vi "Clean Up Actor.vi"(8 "error in (no error)":errorcluster, 11 "Car Position Simulator in":refnum<class "Car Position Simulator.lvclass">) -> (0 "error out":errorcluster, 3 "Car Position Simulator out":refnum<class "Car Position Simulator.lvclass">)   [LabVIEW 2016, in "CLD Exam - Car Wash.lvlib" / "Car Position Simulator.lvclass"]
doc: "--\nCopyright © 2017 Composed SystemsI All rights reserved.\n\nAuthor: Jon McBee <jon.mcbee@composed.io>\n\nThis library is provided \"AS IS\" ,WITHOUT WARRANTIES OR\nCONDITIONS OF ANY KIND, either express or implied.\n\nComposed Systems -- composed.io\n\nStream 0.0.1.1\nJon McBee - Composed Systems\nCopyright (c) 2017, Composed Systems"
uses:
  Car Position Simulator.lvclass
  D:/Repos/Stream/software/Mediator/Classes/Mediated Actor/Mediated Actor.lvclass
  Mediator/Classes/Message Broker Interface/Message Broker Interface.lvclass
  Mediator/Classes/Mediated Synchronous Actor/Mediated Synchronous Actor.lvclass
  Mediator/Classes/Mediated Actor/Mediated Actor.lvclass
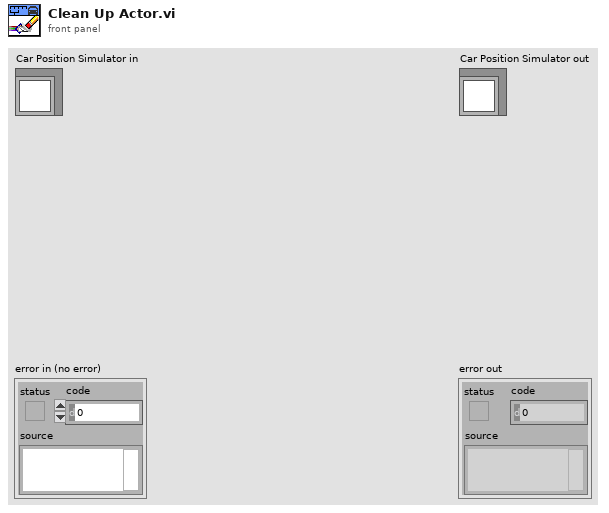
[diagram p1: front panel]
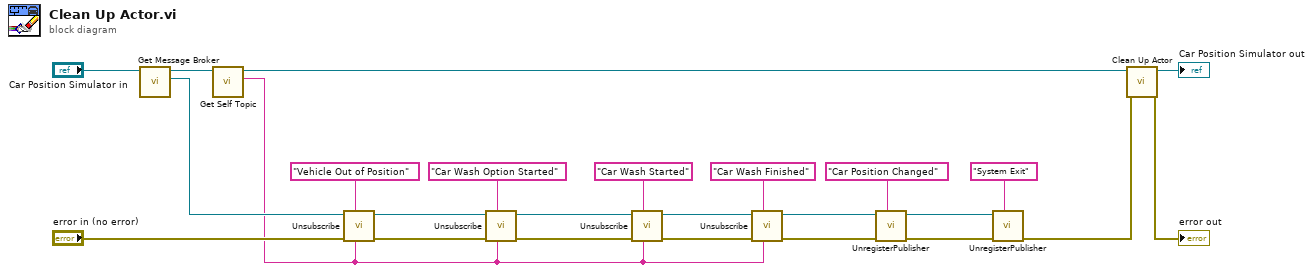
[diagram p0: block diagram]
diagram:
  n1 = call "Get Message Broker.vi"("Mediated Actor in"="Car Position Simulator in") -> ("Message Broker"=w22:refnum<class "Message Broker Interface.lvclass">, "Mediated Actor out"=w23:refnum<class "Car Position Simulator.lvclass">)  [unwired: 9 in]
  n2 = call "Get Self Topic.vi"("Mediated Actor in"=w23) -> ("Topic.Self"=w5:string, "Mediated Actor out"=w19:refnum<class "Car Position Simulator.lvclass">)  [unwired: 9 in]
  n3 = call-dynamic "Unsubscribe.vi"("Subscriber Name"=w5, "Topic Name"="Vehicle Out of Position", "error in (no error)"="error in (no error)", "Message Broker Interface in"=w22) -> ("error out"=w15:errorcluster, "Message Broker Interface out"=w16:refnum<class "Message Broker Interface.lvclass">)  [unwired: 6 in]
  n4 = call-dynamic "Unsubscribe.vi"("Subscriber Name"=w5, "Topic Name"="Car Wash Option Started", "error in (no error)"=w15, "Message Broker Interface in"=w16) -> ("error out"=w7:errorcluster, "Message Broker Interface out"=w9:refnum<class "Message Broker Interface.lvclass">)  [unwired: 6 in]
  n5 = call-dynamic "Unsubscribe.vi"("Subscriber Name"=w5, "Topic Name"="Car Wash Started", "error in (no error)"=w7, "Message Broker Interface in"=w9) -> ("error out"=w6:errorcluster, "Message Broker Interface out"=w8:refnum<class "Message Broker Interface.lvclass">)  [unwired: 6 in]
  n6 = call-dynamic "Unsubscribe.vi"("Subscriber Name"=w5, "Topic Name"="Car Wash Finished", "error in (no error)"=w6, "Message Broker Interface in"=w8) -> ("error out"=w11:errorcluster, "Message Broker Interface out"=w12:refnum<class "Message Broker Interface.lvclass">)  [unwired: 6 in]
  n7 = call-dynamic "UnregisterPublisher.vi"("Topic Name"="Car Position Changed", "error in (no error)"=w11, "Message Broker Interface in"=w12) -> ("error out"=w3:errorcluster, "Message Broker Interface out"=w1:refnum<class "Message Broker Interface.lvclass">)  [unwired: 7 in]
  n8 = call-dynamic "UnregisterPublisher.vi"("Topic Name"="System Exit", "error in (no error)"=w3, "Message Broker Interface in"=w1) -> ("error out"=w2:errorcluster)  [unwired: 7 in, 1 out]
  n9 = call-parent "Clean Up Actor.vi"("error in (no error)"=w2, "Mediated Actor in"=w19) -> ("error out"=→"error out":errorcluster, "Mediated Actor out"=→"Car Position Simulator out":refnum<class "Car Position Simulator.lvclass">)  [unwired: 8 in]
